vi "Kinematics_old.vi"() -> ()   [LabVIEW 2021]
uses:
  <vilib>/express/express arith-compare/Formula/XNode/ExpressFormulaBlockNode.xnode
panel:
  in  "OK Button":bool
  in  "Mass":dbl
  in  "Velocity":dbl
  in  "Angle":dbl
  in  "Height (Initial)":dbl
  in  "Resolution":dbl
  out "XY Graph":cluster{dbl[], dbl[]}[](graph)
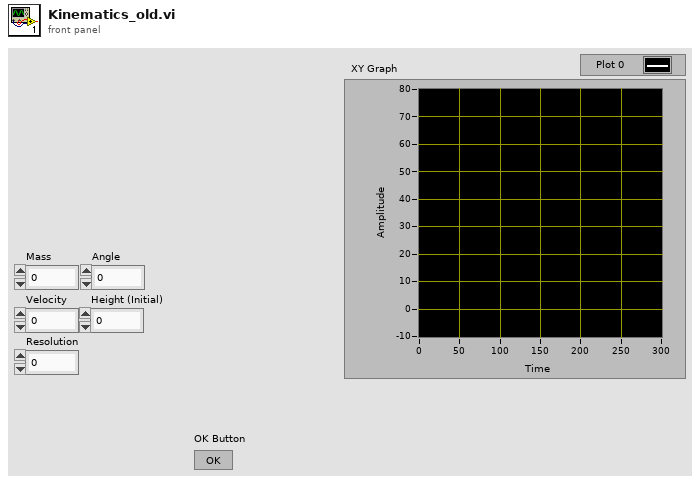
[diagram p1: front panel]
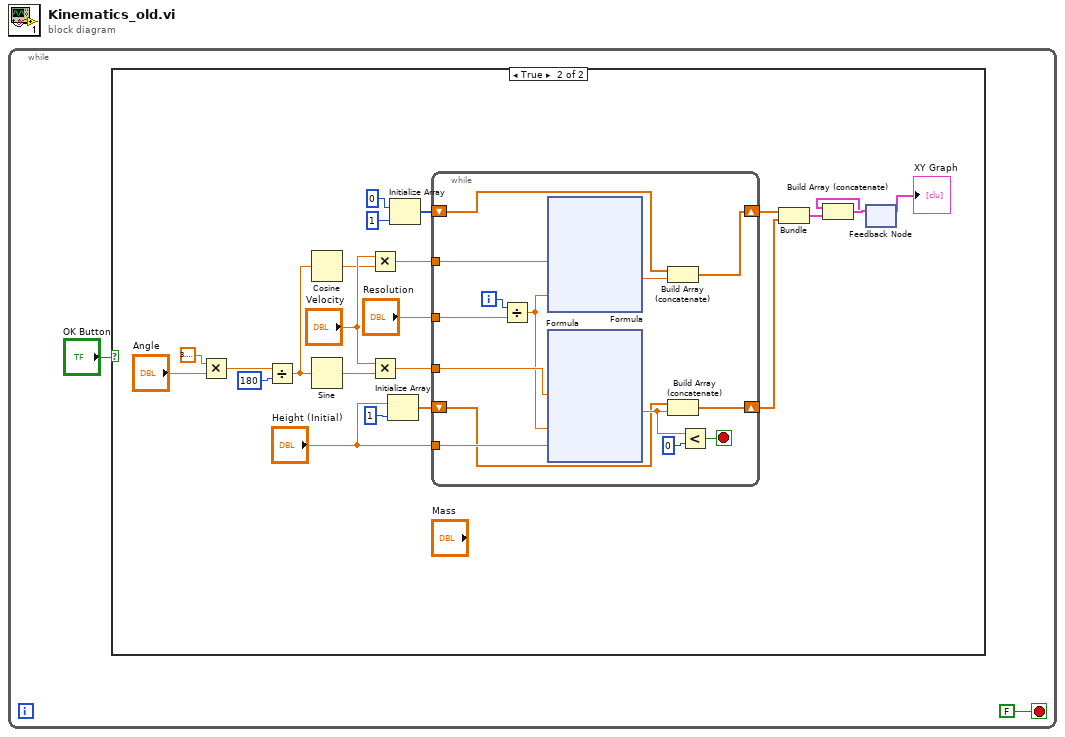
[diagram p0: block diagram]
diagram:
  n1 = while {
    stop <- FALSE stop-if-true
    n2 = case shown="True" "OK Button" {
      frame False {
      }
      frame True {
        n3 = Multiply(x=3.141592653589793, y="Angle") -> (x*y=w22:dbl)
        n4 = Divide(x=w22, y=180) -> (x/y=w20:dbl)
        n5 = Cosine(x=w20) -> (cos(x)=w16:dbl)
        n6 = Sine(x=w20) -> (sin(x)=w19:dbl)
        n7 = Multiply(x="Velocity", y=w16) -> (x*y=w15:dbl)
        n8 = Multiply(x="Velocity", y=w19) -> (x*y=w18:dbl)
        n9 = Initialize Array("Height (Initial)", 1) -> (w8:dbl[])
        n10 = Initialize Array(0, 1) -> (w5:i32[])
        n11 = while {
          tunnel: w18 -> [w35]
          tunnel: w15 -> [w36]
          tunnel: "Height (Initial)" -> [w33]
          tunnel: "Resolution" -> [w37]
          shift-right: [w27] -> w12
          shift-left: w8 -> [w25]
          shift-right: [w28] -> w13
          shift-left: w5 -> [w26]
          i -> [w38]
          stop <- w31 stop-if-true
          n12 = Divide(x=w38, y=w37) -> (x/y=w34:dbl)
          n13 = xnode "Formula"("V_X"=w36, "T"=w34) -> ("Result"=w29:dbl)  [unwired: 1 in, 1 out]
          n14 = xnode "Formula"("V_Y"=w35, "T"=w34, "Y_I"=w33) -> ("Result"=w30:dbl)  [unwired: 1 in, 1 out]
          n15 = Build Array (concatenate)(w26, w29) -> (w28:dbl[])
          n16 = Build Array (concatenate)(w25, w30) -> (w27:dbl[])
          n17 = Less?(x=w30, y=0) -> (x < y?=w31:bool)
        }
        n18 = Bundle(w13, w12) -> (w11:cluster{dbl[], dbl[]})  [unwired: 1 in]
        n19 = feedback #1() -> (w3:cluster{dbl[], dbl[]}[])  [unwired: 1 in]
        "XY Graph" <- w3
        n20 = Build Array (concatenate)(w3, w11) -> (w4:cluster{dbl[], dbl[]}[])
        n21 = feedback-in #1(w4) -> ()
      }
    }
  }
